vi "Add ResMag Analog Channels FXP.vi"(11 "Array in":T1=[0.0, 0.0, 0.0, 0.0, 0.0, 0.0, 0.0, 0.0, 0.0, 0.0, 0.0, 0.0, 0.0, 0.0, 0.0, 0.0, 0.0, 0.0, 0.0, 0.0, 0.0, 0.0, 0.0, 0.0, 0.0, 0.0, 0.0, 0.0, 0.0, 0.0, 0.0, 0.0, 0.0, 0.0, 0.0, 0.0, 0.0, 0.0]) -> (3 "Array out":T2)   [LabVIEW 2018]
doc: "Author: Scott Hannahs <sth@magnet.fsu.edu>\nCopyright 2018 Florida State University, All rights reserved."
uses:
  SCH Data Controls/SCH All FXP Data.ctl
  SCH Data Controls/SCH Raw Offset Data.ctl
  <vilib>/rvi/eio/common/nirviEmuTemplateMethod_errors.vi
  <vilib>/rvi/FXPMathLib/FxpInterpret/XNode/nifxpmath_Interpret.xnode
  <vilib>/eio/EIONode/EIONode.xnode
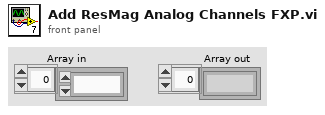
[diagram p1: front panel]
types:
  T1 = typedef "SCH Raw Offset Data.ctl" = fxp<+/-,17,17>[]
  T2 = typedef "SCH All FXP Data.ctl" = fxp<+/-,19,5>[]
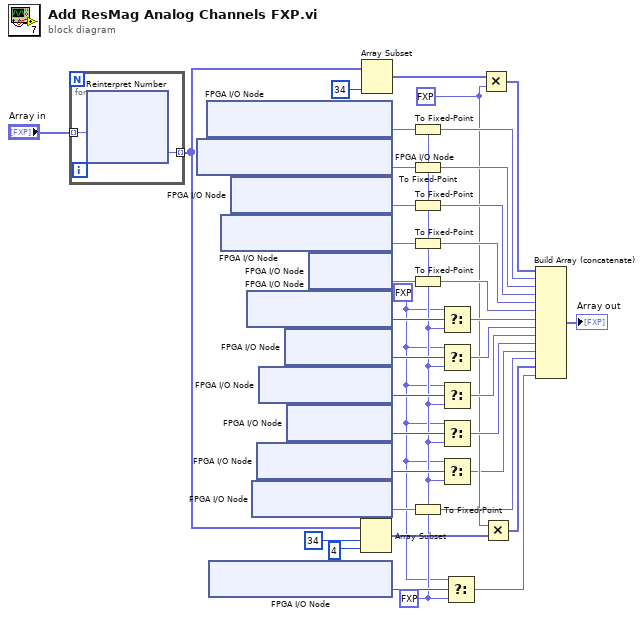
[diagram p0: block diagram]
diagram:
  w2 = fxp<+/-,19,5> 0.0 ("fixed-point type")
  w8 = fxp<+,3,4> 10.0 ("fixed-point type")
  w1 = fxp<+/-,19,5> 1.0 ("fixed-point type")
  n1 = for {
    tunnel: "Array in" -> [w39] mode=indexing
    tunnel: [w38] -> w4 mode=indexing
    n2 = xnode "Reinterpret Number"("x"=w39) -> ("y"=w38:fxp<+/-,17,2>)
  }
  n3 = xnode "FPGA I/O Node"() -> ("Resistive Outlet Temperature"=w18:fxp<+/-,24,5>)  [unwired: 1 in, 1 out]
  n4 = xnode "FPGA I/O Node"() -> ("Resistive Inlet Temperature"=w16:fxp<+/-,24,5>)  [unwired: 1 in, 1 out]
  n5 = xnode "FPGA I/O Node"() -> ("SCHMPS#2 Breaker Enable"=w6:bool)  [unwired: 1 in, 1 out]
  n6 = xnode "FPGA I/O Node"() -> ("Resistive Outlet Pressure"=w22:fxp<+/-,24,5>)  [unwired: 1 in, 1 out]
  n7 = xnode "FPGA I/O Node"() -> ("Resistive Inlet Pressure"=w20:fxp<+/-,24,5>)  [unwired: 1 in, 1 out]
  n8 = xnode "FPGA I/O Node"() -> ("Watchdog Timer In"=w35:bool)  [unwired: 1 in, 1 out]
  n9 = xnode "FPGA I/O Node"() -> ("Bore Tube Voltage"=w14:fxp<+/-,24,5>)  [unwired: 1 in, 1 out]
  n10 = xnode "FPGA I/O Node"() -> ("Watchdog Trip In"=w34:bool)  [unwired: 1 in, 1 out]
  n11 = xnode "FPGA I/O Node"() -> ("Breaker Enable In"=w37:bool)  [unwired: 1 in, 1 out]
  n12 = xnode "FPGA I/O Node"() -> ("PS Enable In"=w36:bool)  [unwired: 1 in, 1 out]
  n13 = xnode "FPGA I/O Node"() -> ("Cell Fault In"=w30:bool)  [unwired: 1 in, 1 out]
  n14 = xnode "FPGA I/O Node"() -> ("Current"=w24:fxp<+/-,24,5>)  [unwired: 1 in, 1 out]
  n15 = Array Subset(array=w4, index=34 ("length"), length=4) -> (w12:fxp<+/-,17,2>[])
  n16 = Array Subset(array=w4, length=34) -> (w13:fxp<+/-,17,2>[])  [unwired: 1 in]
  n17 = To Fixed-Point(fixed-point type=w2, number=w16) -> (fixed-point=w15:fxp<+/-,19,5>)
  n18 = To Fixed-Point(fixed-point type=w2, number=w18) -> (fixed-point=w17:fxp<+/-,19,5>)
  n19 = To Fixed-Point(fixed-point type=w2, number=w20) -> (fixed-point=w19:fxp<+/-,19,5>)
  n20 = To Fixed-Point(fixed-point type=w2, number=w22) -> (fixed-point=w21:fxp<+/-,19,5>)
  n21 = To Fixed-Point(fixed-point type=w2, number=w24) -> (fixed-point=w23:fxp<+/-,19,5>)
  n22 = To Fixed-Point(fixed-point type=w2, number=w14) -> (fixed-point=w11:fxp<+/-,19,5>)
  n23 = Select(t=w1, s=w35, f=w2) -> (s? t:f=w28:fxp<+/-,19,5>)
  n24 = Select(t=w1, s=w36, f=w2) -> (s? t:f=w25:fxp<+/-,19,5>)
  n25 = Select(t=w1, s=w37, f=w2) -> (s? t:f=w27:fxp<+/-,19,5>)
  n26 = Select(t=w1, s=w30, f=w2) -> (s? t:f=w26:fxp<+/-,19,5>)
  n27 = Select(t=w1, s=w34, f=w2) -> (s? t:f=w3:fxp<+/-,19,5>)
  n28 = Select(t=w1, s=w6, f=w2) -> (s? t:f=w7:fxp<+/-,19,5>)
  n29 = Multiply(x=w13, y=w8) -> (x*y=w10:fxp<+/-,19,5>[])
  n30 = Multiply(x=w8, y=w12) -> (x*y=w9:fxp<+/-,19,5>[])
  n31 = Build Array (concatenate)(w10, w15, w17, w19, w21, w23, w28, w25, w27, w26, w3, w11, w9, w7) -> (→"Array out":fxp<+/-,19,5>[])
